vi "General_SimpleMessage_CT.vi"(10 "Message":string) -> (2 "Command":string)   [LabVIEW 2017]
uses:
  sobot structures/SoBot_CommandTypes.ctl
  sobot structures/General_Command.ctl
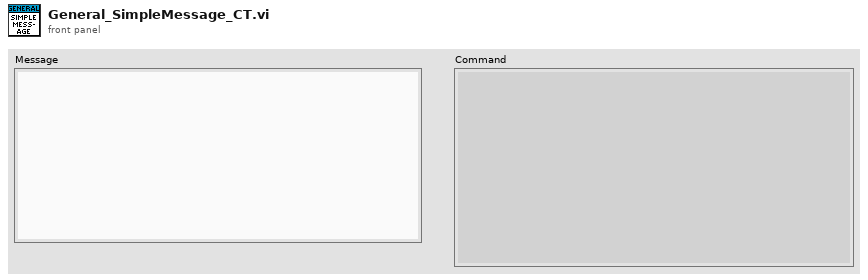
[diagram p1: front panel]
types:
  T1 = typedef "General_Command.ctl" = enum16{"General_Stop", "General_StartSobotAutomatic", "General_StopSobotAutomatic", "General_TransferPoint", "General_Initialize", "General_SimpleMessage", "General_Ping"}
  T2 = typedef "SoBot_CommandTypes.ctl" = enum16{"General_Command", "XY_Command", "Z_Command", "Plattform_Command"}
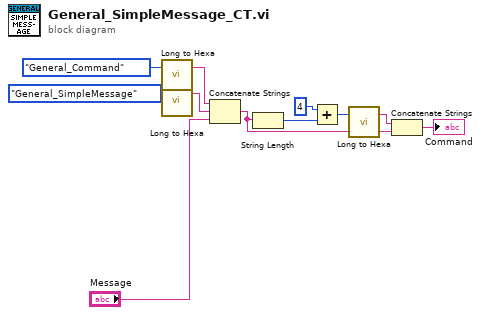
[diagram p0: block diagram]
diagram:
  n1 = call "Long to Hexa.vi"("Long"=SoBot_CommandTypes."General_Command" ("SoBot_CommandTypes")) -> ("Hexa"=w11:string)  [unwired: 2 in]
  n2 = call "Long to Hexa.vi"("Long"=General_Command."General_SimpleMessage" ("General_Command")) -> ("Hexa"=w10:string)  [unwired: 2 in]
  n3 = Concatenate Strings(w11, w10, "Message") -> (w5:string)
  n4 = String Length(string=w5) -> (length=w9:i32)
  n5 = Add(x=4, y=w9) -> (x+y=w7:i32)
  n6 = call "Long to Hexa.vi"("Long"=w7) -> ("Hexa"=w6:string)  [unwired: 2 in]
  n7 = Concatenate Strings(w6, w5) -> (→"Command":string)
